vi "Load LLB Mouse.vi"(11 "Mouse LLB":path) -> (0 "error out":errorcluster, 2 "Name":string, 3 "Mouse":refnum<class "Mouse.lvclass">)   [LabVIEW 2020, in "App.lvlib" / "MazeUI.lvclass"]
uses:
  MazeUI.lvclass
  Maze/Mouse/Mouse.lvclass
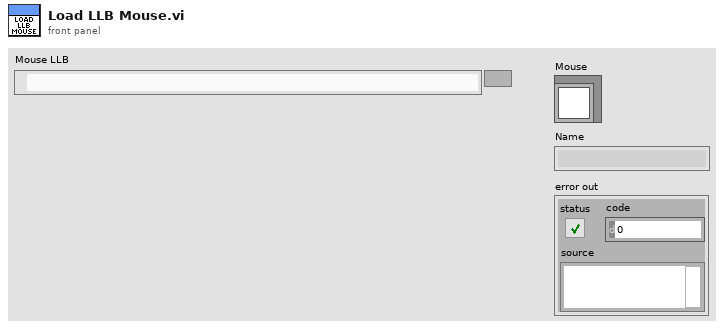
[diagram p1: front panel]
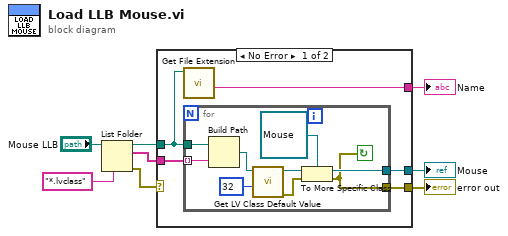
[diagram p0: block diagram]
diagram:
  n1 = List Folder(path="Mouse LLB", pattern="*.lvclass") -> (path out=w5:path, filenames=w6:string[], error out=w4:errorcluster)  [unwired: 2 in, 1 out]
  n2 = case shown="No Error" w4 {
    selector: w4 -> [_ w23]
    tunnel: [w13 _] -> w2
    tunnel: [w12 w23] -> w3
    tunnel: w6 -> [w11 _]
    tunnel: w5 -> [w10 _]
    tunnel: [w9 _] -> w1
    frame No Error {
      n3 = call <vilib>:"Get File Extension.vi"("file"=w10) -> ("filename without extension"=w9:string)  [unwired: 6 in, 4 out]
      n4 = for {
        tunnel: [w21] -> w13
        tunnel: [w19] -> w12
        tunnel: w10 -> [w18]
        tunnel: w11 -> [w17] mode=indexing
        stop <- w19 continue-if-true
        n5 = Build Path(base path=w18, name or relative path=w17) -> (appended path=w14:path)
        n6 = call <vilib>:"Get LV Class Default Value.vi"("options"=u32 32, "class path"=w14) -> ("error out"=w15:errorcluster, "object"=w16:refnum<class>)  [unwired: 8 in]
        n7 = To More Specific Class(target class=refnum<class "Mouse.lvclass"> refnum ("Maze.lvlib:Mouse.lvclass"), reference=w16, error in=w15) -> (specific class reference=w21:refnum<class "Mouse.lvclass">, error out=w19:errorcluster)
      }
    }
    frame Error {
    }
  }
  "error out" <- w3
  "Mouse" <- w2
  "Name" <- w1
